vi "FBG_calibration.vi"() -> ()   [LabVIEW 2013]
uses:
  <vilib>/Platform/TimedLoop/XDataNode/XDataNode.xnode
  <vilib>/Platform/TimedLoop/XDataNode/nitl_modes.ctl
  <vilib>/Platform/TimedLoop/XDataNode/XDNodeRunTimeDep.lvlib
  <vilib>/Platform/TimedLoop/XDataNode/wakeup.ctl
  <vilib>/Platform/TimedLoop/XDataNode/timing_clust.ctl
  host/ltrace_index.ctl
  <vilib>/Analysis/6fits.llb/Curve Fitting Criteria.ctl
  <vilib>/Analysis/NI_AALPro.lvlib
  <vilib>/Analysis/Matrix/NI_Matrix.lvlib
  <vilib>/Analysis/Matrix/Numeric/Conversions/Matrix To Array - RM.vi
  <vilib>/Analysis/NI_AALBase.lvlib
  <vilib>/Analysis/baseanly.llb/Real A x B.vi
  testing/probe_point.ctl
  testing/Trace controls.ctl
  testing/status_flag.ctl
  testing/flag_selector.ctl
  testing/pose_source.ctl
  testing/pose_selector.ctl
  testing/pose_relative_to.ctl
panel:
  out "FBG and Tip Compare":cluster{"A x B":dbl[], "A x B":dbl[]}[](graph)
  out "Difference (deg)":dbl format="%#_3p"
  out "Difference (rad)":dbl
  out "FBG Angle (rad)":dbl format="%#_3p"
  out "FBG Angle (deg)":dbl format="%#_3p"
  out "Tip Angle (deg)":dbl format="%#_3p"
  out "Tip Angle (rad)":dbl format="%#_3p"
  out "FBG Trace":cluster{"Y":sgl[], "Best Linear Fit":dbl[]}[](graph)
  out "Tip Trace":cluster{"Y":sgl[], "Best Linear Fit":dbl[]}[](graph)
  in  "Line fit":bool
  out "Cursor time":timestamp
  out "Trace display":T1(graph)
  out "Progress":u8(slide) scale=0.0..100.0
  in  "Save trace":bool
  in  "Output path":path
  out "Sequence error":bool
  out "Out of order":i32
  out "Missing":i32
  out "Chunk binary data file":path caption="selected path"
  out "File exists":bool
  in  "Input file":path
  in  "stop":bool
  in  "Reference hold":bool
  in  "Pose selectors":T2[](array[typedef])
  in  "Flag selectors":T5[](array[typedef])=[{"Flag"=enum."Cancellation", "Select"=TRUE}, {"Flag"=enum."Goal filter", "Select"=TRUE}, {"Flag"=enum."Valid position", "Select"=TRUE}, {"Flag"=enum."Velocity limiting", "Select"=TRUE}]
  in  "Decimate":i32=1 min=1 max=999 step=1
  out "2D position":cluster{"X":sgl[], "Y":sgl[]}[](graph)
  in  "Trace controls":T7[](array[typedef])=[{"+ stim"=FALSE, "Relative"=FALSE, "Scale"=enum."1X", "Probe point"=enum."Null pos (tip)", "XYZ selector"={"Boolean"=FALSE, "Boolean 2"=FALSE, "Boolean 3"=TRUE}, "To tip"=TRUE}, {"+ stim"=FALSE, "Relative"=FALSE, "Scale"=enum."1X", "Probe point"=enum."Goal (tip)", "XYZ selector"={"Boolean"=FALSE, "Boolean 2"=FALSE, "Boolean 3"=TRUE}, "To tip"=TRUE}, {"+ stim"=FALSE, "Relative"=FALSE, "Scale"=enum."1X", "Probe point"=enum."Position (tip)", "XYZ selector"={"Boolean"=FALSE, "Boolean 2"=FALSE, "Boolean 3"=TRUE}, "To tip"=TRUE}, {"+ stim"=FALSE, "Relative"=FALSE, "Scale"=enum."1X", "Probe point"=enum."Position (tip)", "XYZ selector"={"Boolean"=FALSE, "Boolean 2"=FALSE, "Boolean 3"=FALSE}, "To tip"=FALSE}]
  # "Trace Display"
  # "Radians"
  # "Degrees"
  # "Tip Angle"
  # "FBG Angle"
  # "Difference"
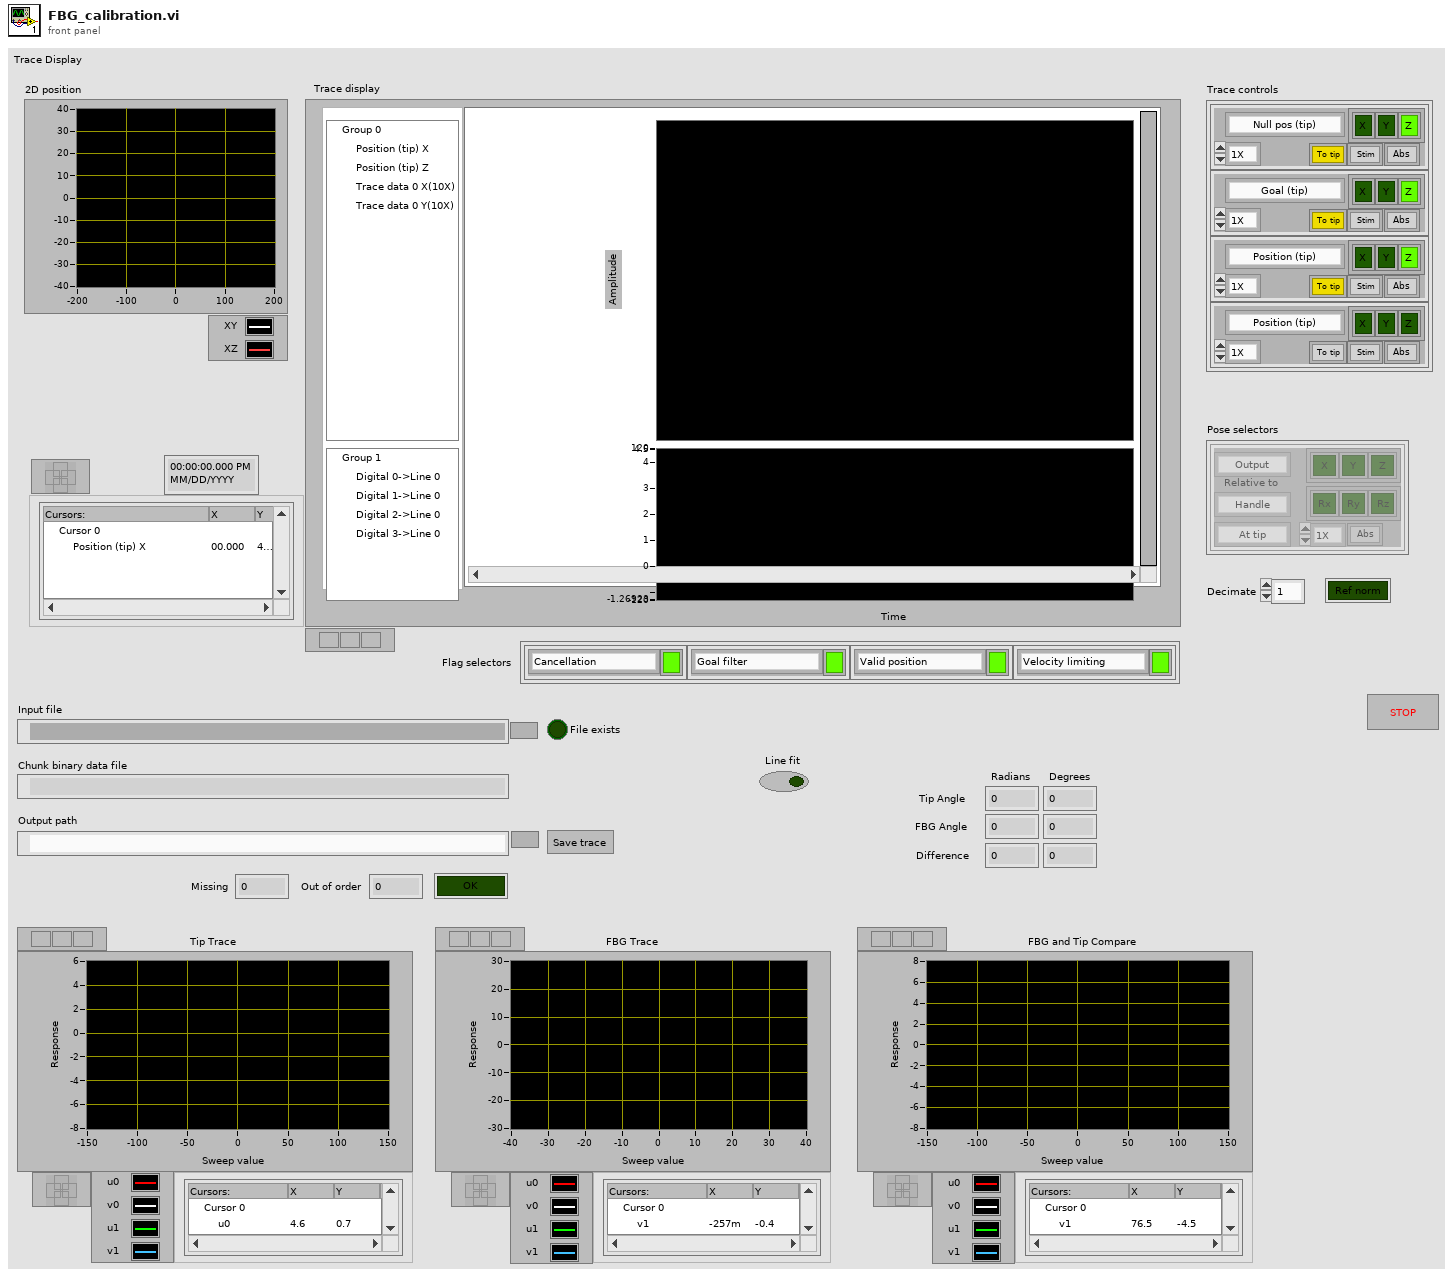
[diagram p1: front panel]
types:
  T1 = cluster{"Waveforms out":waveform(sgl)[], "Digital waveforms":digitalwaveform[]}
  T2 = typedef "pose_selector.ctl" = cluster{"Scale":enum16{"1X", "10X", "100X", "1KX", "10KX"}, "Source":T3, "XYZ selector":cluster{"Boolean":bool, "Boolean 2":bool, "Boolean 3":bool}, "RPY selector":cluster{"Boolean":bool, "Boolean 2":bool, "Boolean 3":bool}, "Relative to":T4, "Relative":bool, "Translate":enum16{"At tip", "At RCM", "At KC", "At origin"}}
  T3 = typedef "pose_source.ctl" = enum16{"Output", "Handle", "Handle KF", "Goal", "Absolute"}
  T4 = typedef "pose_relative_to.ctl" = enum16{"Output", "Handle", "Handle KF", "Goal", "Absolute", "Trace start"}
  T5 = typedef "flag_selector.ctl" = cluster{"Flag":T6, "Select":bool}
  T6 = typedef "status_flag.ctl" = enum16{"Cancellation", "Goal filter", "Valid position", "Goal saturation tip", "Goal saturation RCM", "Goal circle saturation", "Position saturation", "Output saturation", "Acceleration limiting", "Finished late", "Stimulus increasing", "Integral error saturation", "Velocity limiting", "Log warning", "Log error", "Link KF degraded"}
  T7 = typedef "Trace controls.ctl" = cluster{"+ stim":bool, "Relative":bool, "Scale":enum16{"1X", "10X", "100X", "1KX", "10KX"}, "Probe point":T8, "XYZ selector":cluster{"Boolean":bool, "Boolean 2":bool, "Boolean 3":bool}, "To tip":bool}
  T8 = typedef "probe_point.ctl" = enum16{"Position (tip)", "Position (RCM)", "Null pos (tip)", "Null pos (RCM)", "V limiter (tip)", "V Limiter (RCM)", "Goal (tip)", "Goal (RCM)", "Link pos 0", "Link pos 1", "KF link pos 0", "KF link pos 1", "Link rate 0", "Link rate 1", "Link residue 0", "Link residue 1", "Link goal 0", "Link goal 1", "Rate limit 0", "Rate limit 1", "Link error 0", "Link error 1", "Controller 0", "Controller 1", "Output 0", "Output 1", "Drive 0", "Drive 1", "Stimulus 0", "Stimulus 1", "Trace data 0", "Trace data 1", "Analog data 0", "Analog data 1", "Status flags", "Light 0", "Light 1", "Light 2", "Light 3", "Light 4", "Light 5", "Goal origin", "Goal rotation 0", "Goal rotation 1", "Goal rotation 2", "Output origin", "Output rotation 0", "Output rotation 1", "Output rotation 2", "Handle origin", "Handle rotation 0", "Handle rotation 1", "Handle rotation 2", "Handle position", "Handle velocity", "Handle acceleration", "Handle angles", "Handle angle rates", "Handle pos residue", "Handle angle residue", "Trace length"}
  T9 = typedef "XDNodeRunTimeDep.lvlib/timing_clust.ctl" = cluster{"Expected End [f-1]":u64, "Actual End [f-1]":u64, "Finished Late? [f-1]":bool, "Expected End [i-1]":u64, "Actual End [i-1]":u64, "Finished Late? [i-1]":bool, "Expected Start [i]":u64, "Actual Start [i]":u64, "Expected Start [f]":u64, "Actual Start [f]":u64, "Source Name":string, "Structure Name":string, "Period":i64, "Deadline":i64, "Offset":i64, "Start":i64, "Priority":i32, "Timeout":i32, "Mode":T10, "Wakeup Reason":T11, "Error":errorcluster, "Source Type":string, "Secondary Source Type":string, "Global End Time":u64, "Global Start Time":u64, "Frame Duration":u64, "Iteration Duration":u64, "Assigned CPU":i32, "I/O Scan Engine Mode":u32}
  T10 = typedef "XDNodeRunTimeDep.lvlib/nitl_modes.ctl" = enum32{"No Change", "Process missed periods, maintain original phase", "Discard missed periods, maintain original phase", "Process missed periods, ignore original phase", "Discard missed periods, ignore original phase"}
  T11 = typedef "XDNodeRunTimeDep.lvlib/wakeup.ctl" = enum32{"Normal", "Aborted", "Asynchronous wakeup", "Timing source error", "Timed loop error", "Timeout"}
  T12 = typedef "ltrace_index.ctl" = cluster{"Timestamp":timestamp, "Offset":i64, "Sequence":u32, "Flags":u32}
  T13 = typedef "NI_AALPro.lvlib/Curve Fitting Criteria.ctl" = u16
  T14 = typedef "NI_Matrix.lvlib/RealMatrix.ctl" = dbl[][]
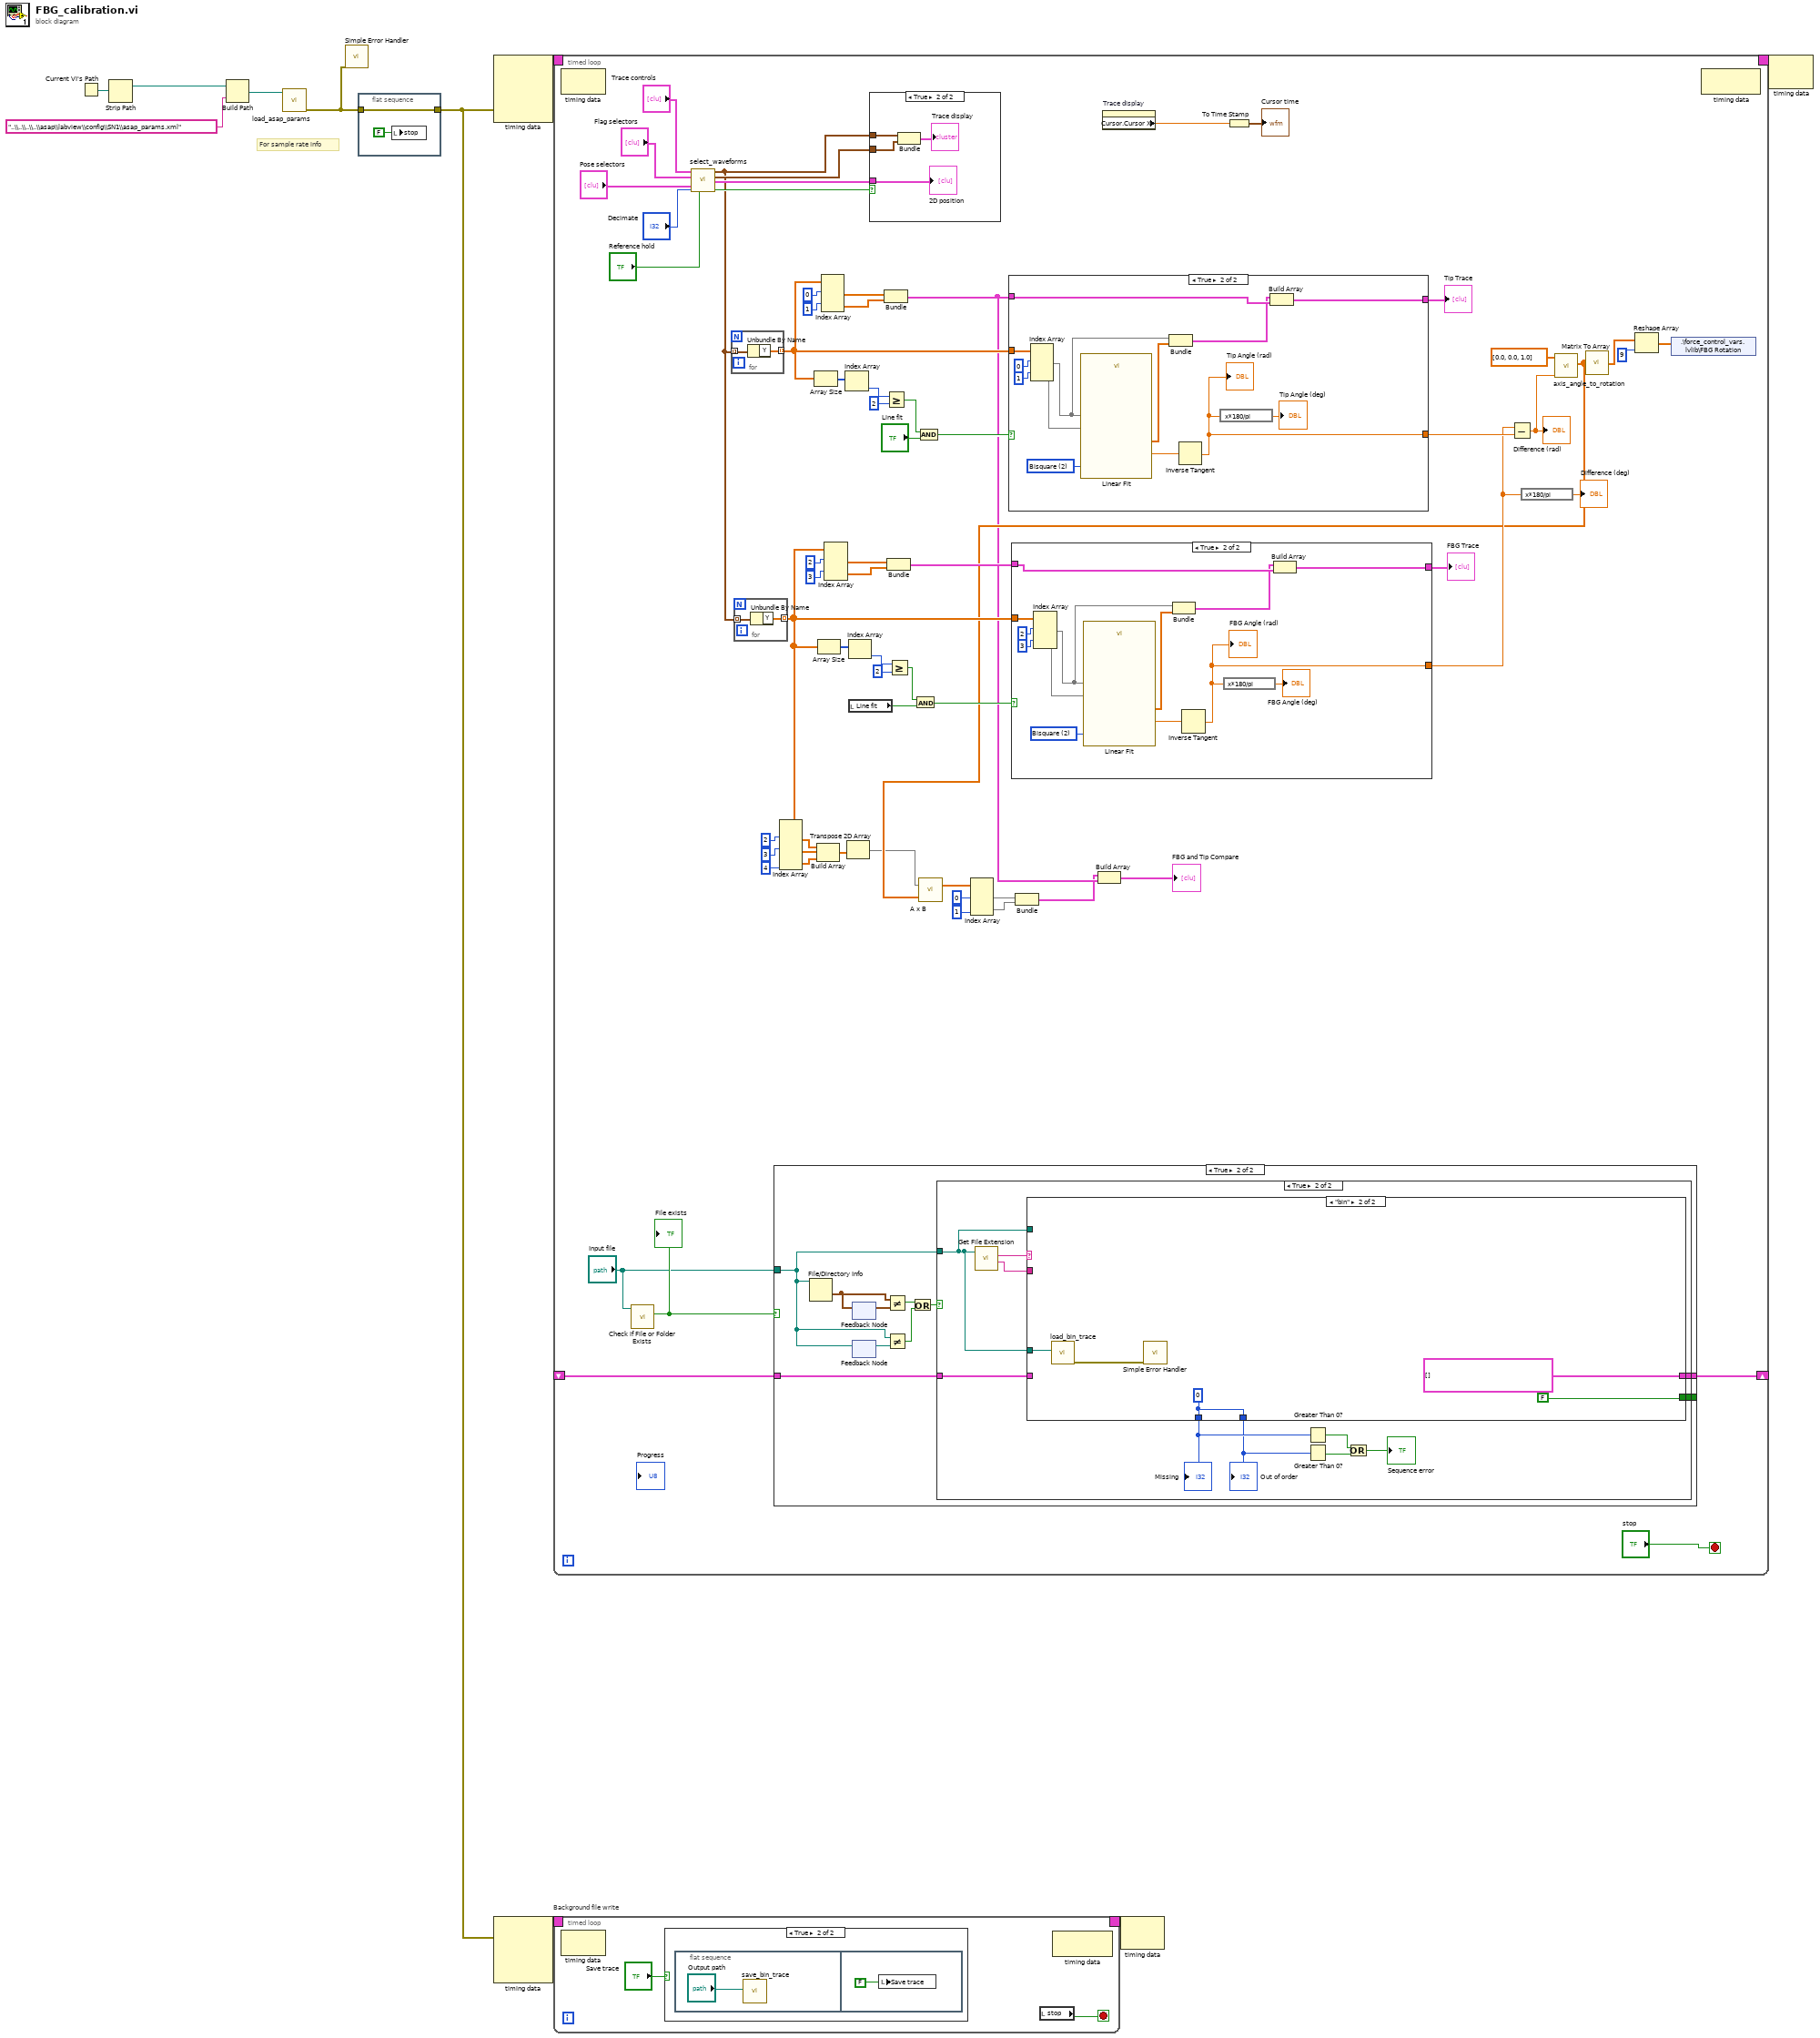
[diagram p0: block diagram]
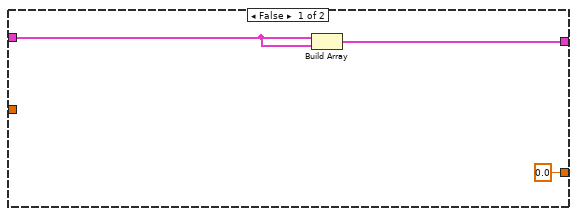
[diagram p3: hidden frame]
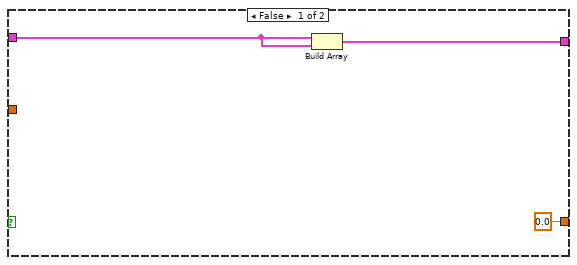
[diagram p4: hidden frame]
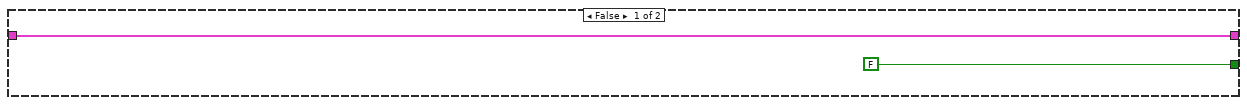
[diagram p5: hidden frame]
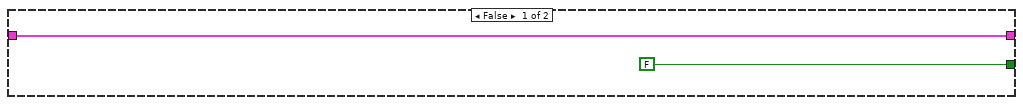
[diagram p6: hidden frame]
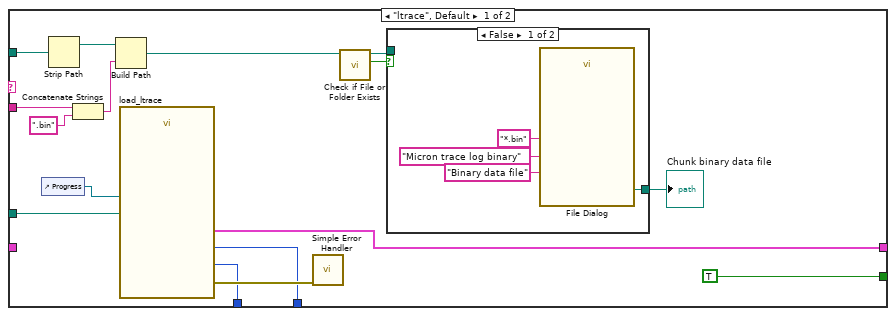
[diagram p7: hidden frame]
diagram:
  # "For sample rate info"
  n1 = Current VI's Path() -> (path=w5:path)
  n2 = Strip Path(path=w5) -> (stripped path=w4:path)  [unwired: 1 out]
  n3 = Build Path(base path=w4, name or relative path="..\\..\\..\\..\\asap\\labview\\config\\SN1\\asap_params.xml") -> (appended path=w2:path)
  n4 = call "load_asap_params.vi"("ASAP params file"=w2) -> ("error out"=w1:errorcluster)  [unwired: 10 in]
  n5 = call <vilib>:"Simple Error Handler.vi"("error in (no error)"=w1) -> ()  [unwired: 4 in, 5 out]
  n6 = flat-sequence {
    tunnel: [w12] -> w6
    tunnel: w1 -> [w12]
    frame #0 {
      n7 = local write "stop"(FALSE ("stop")) -> ()
    }
  }
  n8 = node-c288(w6) -> (w10:T9)  [unwired: 3 in]
  n9 = node-c288(w6) -> (w8:T9)  [unwired: 3 out]
  n10 = timed-loop {
    timing: w10 -> [_]
    timing-out: [_] -> w9
    shift-right: [w66] -> _
    shift-left: _ -> [w67]
    stop <- "stop" stop-if-true
    n11 = node-c288() -> ()  [unwired: 1 in, 1 out]
    n12 = call <vilib>:"Check if File or Folder Exists.vi"("path"="Input file") -> ("file or folder exists?"=w69:bool)  [unwired: 8 in, 2 out]
    "File exists" <- w69
    n13 = call "select_waveforms.vi"("Trace controls"="Trace controls", "Flag selectors"="Flag selectors", "Pose selectors"="Pose selectors", "Decimate"="Decimate", "Reference hold"="Reference hold") -> ("Waveforms out"=w40:waveform(sgl)[], "Digital waveforms"=w75:digitalwaveform[], "XY views"=w76:cluster{"X":sgl[], "Y":sgl[]}[], "New data"=w77:bool)  [unwired: 7 in]
    n14 = for {
      tunnel: w40 -> [w113] mode=indexing
      tunnel: [w114] -> w54 mode=indexing
      n15 = Unbundle By Name(w113) -> ("Y"=w114:sgl[])
    }
    n16 = for {
      tunnel: w40 -> [w95] mode=indexing
      tunnel: [w96] -> w24 mode=indexing
      n17 = Unbundle By Name(w95) -> ("Y"=w96:sgl[])
    }
    n18 = case shown="True" w69 {
      tunnel: "Input file" -> [_ w123]
      tunnel: w67 -> [w116 w119]
      tunnel: [w116 w118] -> w66
      tunnel: [FALSE ("x .or. y?") w117] -> _
      frame False {
      }
      frame True {
        n19 = File/Directory Info(path=w123) -> (last mod=w124:timestamp)  [unwired: 1 in, 6 out]
        n20 = feedback #1() -> (w125:timestamp)  [unwired: 1 in]
        n21 = feedback-in #1(w124) -> ()
        n22 = feedback #2() -> (w126:path)  [unwired: 1 in]
        n23 = feedback-in #2(w123) -> ()
        n24 = Not Equal?(x=w124, y=w125) -> (x != y?=w122:bool)
        n25 = Not Equal?(x=w123, y=w126) -> (x != y?=w121:bool)
        n26 = Or(x=w122, y=w121) -> (x .or. y?=w120:bool)
        n27 = case shown="True" w120 {
          tunnel: w123 -> [_ w129]
          tunnel: w119 -> [w128 w132]
          tunnel: [w128 w131] -> w118
          tunnel: [FALSE ("x .or. y?") w130] -> w117
          frame False {
          }
          frame True {
            n28 = call <vilib>:"Get File Extension.vi"("file"=w129) -> ("filename without extension"=w138:string, "lowercase file extension"=w139:string)  [unwired: 7 in, 2 out]
            n29 = case shown="\"bin\"" w139 {
              tunnel: w129 -> [w155 w165]
              tunnel: w138 -> [w153 _]
              tunnel: [w148 w163] -> w137
              tunnel: [w147 w163] -> w136
              tunnel: w132 -> [_ _]
              tunnel: [w146 T12[] [] ("File index")] -> w131
              tunnel: [TRUE ("x .or. y?") FALSE ("x .or. y?")] -> w130
              tunnel: w129 -> [w144 _]
              frame "ltrace", Default {
                n30 = control-ref of="Progress"() -> (w140:refnum<vi>)
                n31 = Strip Path(path=w144) -> (stripped path=w143:path)  [unwired: 1 out]
                n32 = Concatenate Strings(w153, ".bin" ("string")) -> (w142:string)
                n33 = Build Path(base path=w143, name or relative path=w142) -> (appended path=w141:path)
                n34 = call "load_ltrace.vi"("Progress"=w140, "File path"=w155) -> ("error out"=w149:errorcluster, "File index"=w146:T12[], "Out of order"=w147:i32, "Missing"=w148:i32)  [unwired: 5 in, 1 out]
                n35 = call <vilib>:"Simple Error Handler.vi"("error in (no error)"=w149) -> ()  [unwired: 4 in, 5 out]
                n36 = call <vilib>:"Check if File or Folder Exists.vi"("path"=w141) -> ("file or folder exists?"=w151:bool, "dup path"=w150:path)  [unwired: 8 in, 1 out]
                n37 = case shown="False" w151 {
                  tunnel: [w156 w160] -> w152
                  tunnel: w150 -> [_ w160]
                  frame False {
                    n38 = call "File Dialog"("prompt"="Binary data file", "pattern (all files)"="*.bin", "pattern label"="Micron trace log binary") -> ("selected path"=w156:path)  [unwired: 9 in, 3 out]
                  }
                  frame True {
                  }
                }
                "Chunk binary data file" <- w152
              }
              frame "bin" {
                w163 = 0 ("Missing")
                n39 = call "load_bin_trace.vi"("File path"=w165) -> ("error out"=w164:errorcluster)  [unwired: 9 in, 1 out]
                n40 = call <vilib>:"Simple Error Handler.vi"("error in (no error)"=w164) -> ()  [unwired: 4 in, 5 out]
              }
            }
            "Missing" <- w137
            "Out of order" <- w136
            n41 = Greater Than 0?(x=w137) -> (x > 0?=w135:bool)
            n42 = Greater Than 0?(x=w136) -> (x > 0?=w134:bool)
            n43 = Or(x=w135, y=w134) -> (x .or. y?=→"Sequence error":bool)
          }
        }
      }
    }
    n44 = Index Array(array=w24, index (row) #1=2 ("disabled index (col)"), index (row) #2=3 ("index"), index (row) #3=4 ("index (row)")) -> (element #1=w23:sgl[], element #2=w22:sgl[], element #3=w21:sgl[])  [unwired: 3 in]
    n45 = Array Size(array=w54) -> (size(s)=w60:i32[])
    n46 = Build Array(w23, w22, w21) -> (w18:sgl[][])
    n47 = Array Size(array=w24) -> (size(s)=w43:i32[])
    n48 = Index Array(array=w54, index (row) #1=0 ("disabled index (col)"), index (row) #2=1 ("index")) -> (element #1=w56:sgl[], element #2=w55:sgl[])  [unwired: 2 in]
    n49 = Index Array(array=w24, index (row) #1=2 ("disabled index (col)"), index (row) #2=3 ("index")) -> (element #1=w48:sgl[], element #2=w49:sgl[])  [unwired: 2 in]
    n50 = Index Array(array=w60) -> (element=w59:i32)  [unwired: 1 in]
    n51 = Transpose 2D Array(2D array=w18) -> (transposed array=w17:sgl[][])
    n52 = Index Array(array=w43) -> (element=w44:i32)  [unwired: 1 in]
    n53 = local read "Line fit"() -> (w39:bool)
    n54 = case shown="True" w77 {
      tunnel: w40 -> [_ w168]
      tunnel: w76 -> [_ w169]
      tunnel: w75 -> [_ w167]
      frame False {
      }
      frame True {
        n55 = Bundle("Waveforms out"=w168, "Digital waveforms"=w167) -> (→"Trace display":T1)  [unwired: 1 in]
        "2D position" <- w169
      }
    }
    n56 = Bundle("Y"=w56, "Y"=w55) -> (w14:cluster{"Y":sgl[], "Y":sgl[]})  [unwired: 1 in]
    n57 = Greater Or Equal?(x=w59, y=2) -> (x >= y?=w63:bool)
    n58 = Bundle("Y"=w48, "Y"=w49) -> (w47:cluster{"Y":sgl[], "Y":sgl[]})  [unwired: 1 in]
    n59 = Greater Or Equal?(x=w44, y=2) -> (x >= y?=w41:bool)
    n60 = And(x=w41, y=w39) -> (x .and. y?=w45:bool)
    n61 = And(x=w63, y="Line fit") -> (x .and. y?=w58:bool)
    n62 = case shown="True" w58 {
      tunnel: w54 -> [_ w112]
      tunnel: [w98 w105] -> w57
      tunnel: w14 -> [w99 w102]
      tunnel: [0.0 w100] -> w38
      frame False {
        n63 = Build Array(w99, w99) -> (w98:cluster{"Y":sgl[], "Y":sgl[]}[])
      }
      frame True {
        w111 = T13 2 items=["Least Square", "Least Absolute Residual", "Bisquare"] ("method")
        n64 = Index Array(array=w112, index (row) #1=0 ("disabled index (col)"), index (row) #2=1 ("index (col)")) -> (element #1=w107:sgl[], element #2=w110:sgl[])  [unwired: 2 in]
        n65 = call <vilib>:"Linear Fit.vi"("Y"=w110, "X"=w107, "method"=w111) -> ("Best Linear Fit"=w106:dbl[], "slope"=w109:dbl)  [unwired: 8 in, 3 out]
        n66 = Bundle("Y"=w107, "Best Linear Fit"=w106) -> (w101:cluster{"Y":sgl[], "Best Linear Fit":dbl[]})  [unwired: 1 in]
        n67 = Inverse Tangent(1:w109) -> (0:w100:dbl)
        "Tip Angle (rad)" <- w100
        n68 = expression code="x*180/pi"(w100) -> (→"Tip Angle (deg)":dbl)
        n69 = Build Array(w101, w102) -> (w105:cluster{"Y":sgl[], "Best Linear Fit":dbl[]}[])
      }
    }
    "Tip Trace" <- w57
    n70 = case shown="True" w45 {
      tunnel: w24 -> [_ w94]
      tunnel: [w80 w87] -> w46
      tunnel: w47 -> [w81 w84]
      tunnel: [0.0 w82] -> w36
      frame False {
        n71 = Build Array(w81, w81) -> (w80:cluster{"Y":sgl[], "Y":sgl[]}[])
      }
      frame True {
        w93 = T13 2 items=["Least Square", "Least Absolute Residual", "Bisquare"] ("method")
        n72 = Index Array(array=w94, index (row) #1=2 ("disabled index (col)"), index (row) #2=3 ("index (col)")) -> (element #1=w89:sgl[], element #2=w92:sgl[])  [unwired: 2 in]
        n73 = call <vilib>:"Linear Fit.vi"("Y"=w92, "X"=w89, "method"=w93) -> ("Best Linear Fit"=w88:dbl[], "slope"=w91:dbl)  [unwired: 8 in, 3 out]
        n74 = Bundle("Y"=w89, "Best Linear Fit"=w88) -> (w83:cluster{"Y":sgl[], "Best Linear Fit":dbl[]})  [unwired: 1 in]
        n75 = Inverse Tangent(1:w91) -> (0:w82:dbl)
        "FBG Angle (rad)" <- w82
        n76 = expression code="x*180/pi"(w82) -> (→"FBG Angle (deg)":dbl)
        n77 = Build Array(w83, w84) -> (w87:cluster{"Y":sgl[], "Best Linear Fit":dbl[]}[])
      }
    }
    "FBG Trace" <- w46
    n78 = property on="Trace display" class="MixedGraph (strict)"() -> ("Cursor.Cursor X"=w65:dbl)  [unwired: 2 in, 2 out]
    n79 = To Time Stamp(1:w65) -> (0:→"Cursor time":timestamp)
    n80 = Subtract(x=w36, y=w38) -> (x-y=w35:dbl)
    "Difference (rad)" <- w35
    n81 = expression code="x*180/pi"(w36) -> (→"Difference (deg)":dbl)
    n82 = call "axis_angle_to_rotation.vi"("Angle"=w35, "Axis"=dbl[] [0.0, 0.0, 1.0]) -> ("Rotation"=w19:T14)  [unwired: 9 in]
    n83 = call-poly <vilib>:"A x B.vi"("B"=w19, "A"=w17) -> ("A x B"=w28:T14)  [unwired: 1 out]
    n84 = Index Array(array=w28, index (col) #1=0 ("disabled index (col)"), index (col) #2=1 ("index")) -> (element #1=w30:dbl[], element #2=w29:dbl[])  [unwired: 2 in]
    n85 = Bundle("A x B"=w30, "A x B"=w29) -> (w13:cluster{"A x B":dbl[], "A x B":dbl[]})  [unwired: 1 in]
    n86 = Build Array(w13, w14) -> (→"FBG and Tip Compare":cluster{"A x B":dbl[], "A x B":dbl[]}[])
    n87 = call-poly <vilib>:"Matrix To Array.vi"("Real Matrix"=w19) -> ("Real 2D Array"=w33:dbl[][])
    n88 = Reshape Array(w33, 9 ("dimension size")) -> (w31:dbl[])
    n89 = shared-variable ".\\force_control_vars.lvlib\\FBG Rotation"(w31) -> ()  [unwired: 1 in, 1 out]
    n90 = node-c288() -> ()  [unwired: 1 in, 1 out]
  }
  n91 = timed-loop "Background file write" {
    timing: w8 -> [_]
    timing-out: [_] -> w7
    stop <- w172 stop-if-true
    n92 = node-c288() -> ()  [unwired: 2 out]
    n93 = case shown="True" "Save trace" {
      frame False {
      }
      frame True {
        n94 = flat-sequence {
          frame #0 {
            n95 = call "save_bin_trace.vi"("File path"="Output path") -> ()  [unwired: 1 in, 10 out]
          }
          frame #1 {
            n96 = local write "Save trace"(FALSE ("Save trace")) -> ()
          }
        }
      }
    }
    n97 = local read "stop"() -> (w172:bool)
    n98 = node-c288() -> ()  [unwired: 2 out]
  }
  n99 = node-c288(w7) -> ()  [unwired: 1 out]
  n100 = node-c288(w9) -> ()  [unwired: 1 out]
